vi "Open Session.vi"(0 "instruction target":refnum<class "niInstr Instruction Target v1 Host.lvclass">, 5 "parent context":refnum<class "niInstr Instruction Framework Context v1 Host.lvclass">, 7 "channel instance":u8, 11 "error in":errorcluster, 12 "select session":refnum<class "niHighSpeedSerial Eye Scan Single Point v1 Host.lvclass">) -> (4 "eye scan single point out":refnum<class "niHighSpeedSerial Eye Scan Single Point v1 Host.lvclass">, 15 "error out":errorcluster)   [LabVIEW 2016, in "niHighSpeedSerial Eye Scan Single Point v1 Host.lvclass"]
doc: "Opens a session to the Single Point Eye Scan class.\n\n<B>Input Parameters</B>\n\n<B>instruction target</B> is the instruction target to use when communicating with the FPGA.\n\n<B>parent context</B> is the context of the parent instance. In most cases you can wire a default value.\n\n<B>channel instance</B> The instance of the channel to be used.\n\n<B>error in</B> describes error conditions that occur before this node runs. This input provides standard 'error in' functionality.\n\n<B>Output Parameters</B>\n\n<B>eye scan single point out</B> passes a reference to your session to the next VI.\n\n<B>error out</B> contains error information. This output provides standard 'error out' functionality."
uses:
  <instrlib>/niHighSpeedSerial/Eye Scan/v1/Host/Impl/Single Point/niHighSpeedSerial Eye Scan Single Point v1 Host.lvclass
  <instrlib>/_niInstr/Instruction Framework/v1/Host/Instruction Target/niInstr Instruction Target v1 Host.lvclass
  <instrlib>/_niInstr/Instruction Framework/v1/Host/Instruction Framework Context/niInstr Instruction Framework Context v1 Host.lvclass
  <instrlib>/niHighSpeedSerial/Eye Scan/v1/Host/Impl/Single Point/Private/Private Data.ctl
  <instrlib>/niHighSpeedSerial/Register Maps/Xilinx/v1/Host/GTX2_CHANNEL v1 Host.llb/GTX2_CHANNEL Register Map.lvclass
  <instrlib>/niHighSpeedSerial/Eye Scan/v1/Host/Impl/Single Point/Private/Channel Measure State.ctl
  <instrlib>/niHighSpeedSerial/Eye Scan/v1/Host/Common/Public/Data Width.ctl
  <instrlib>/niHighSpeedSerial/Eye Scan/v1/Host/Common/Public/Point Offsets.ctl
  <instrlib>/niHighSpeedSerial/Register Maps/Xilinx/v1/Host/GTX2_CHANNEL v1 Host.llb/ESVertOffsetSign.ctl
  <instrlib>/niHighSpeedSerial/Eye Scan/v1/Host/Impl/Single Point/Private/Counts.ctl
  <instrlib>/niHighSpeedSerial/Register Maps/Xilinx/v1/Host/GTX2_CHANNEL v1 Host.llb/GTX2_CHANNEL Register Map.lvclass/GTX2_CHANNEL Register Map.ctl
  <instrlib>/niHighSpeedSerial/Eye Scan/v1/Host/Impl/Single Point/niHighSpeedSerial Eye Scan Single Point v1 Host.lvclass/niHighSpeedSerial Eye Scan Single Point v1 Host.ctl
  <instrlib>/_niInstr/Instruction Framework/v1/Host/Subsystem Map/Private/Lookup Single Context.vi
  <instrlib>/_niInstr/Instruction Framework/v1/Host/Subsystem Map/niInstr Subsystem Map v1 Host.lvclass
  <instrlib>/niHighSpeedSerial/Eye Scan/v1/Host/Common/niHighSpeedSerial Eye Scan Common v1 Host.lvlib
  <instrlib>/niHighSpeedSerial/Register Maps/Xilinx/v1/Host/GTX2_CHANNEL v1 Host.llb/GTX2_CHANNEL v1 Host.lvlib
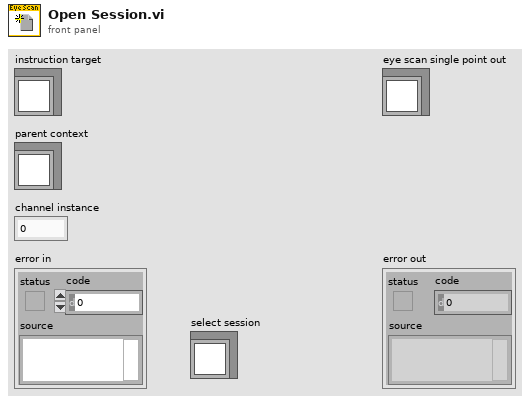
[diagram p1: front panel]
types:
  T1 = typedef "GTX2_CHANNEL v1 Host.lvlib/ESVertOffsetSign.ctl" = enum8{"Positive", "Negative"}
  T2 = typedef "niHighSpeedSerial Eye Scan Common v1 Host.lvlib/Data Width.ctl" = enum16{"16 Bit", "20 Bit", "32 Bit", "40 Bit"}
  T3 = typedef "niHighSpeedSerial Eye Scan Common v1 Host.lvlib/Point Offsets.ctl" = cluster{"horizontal offset":i16, "vertical offset":i8}
  T4 = typedef "niHighSpeedSerial Eye Scan Single Point v1 Host.lvclass/Channel Measure State.ctl" = enum16{"Uninitialized", "Initialized", "Ready", "Request", "Wait", "Read", "Process", "Finished"}
  T5 = typedef "niHighSpeedSerial Eye Scan Single Point v1 Host.lvclass/Private Data.ctl" = cluster{"GTX2_CHANNEL register map":refnum<class "GTX2_CHANNEL Register Map.lvclass">, "instruction target":refnum<class "niInstr Instruction Target v1 Host.lvclass">, "channel measure state":T4, "in DFE mode?":bool, "prescale":u8, "rx internal data width":T2, "active point":T3, "ut sign":T1, "positive counts":T6, "negative counts":T6}
  T6 = typedef "niHighSpeedSerial Eye Scan Single Point v1 Host.lvclass/Counts.ctl" = cluster{"sample count":u64, "error count":u16}
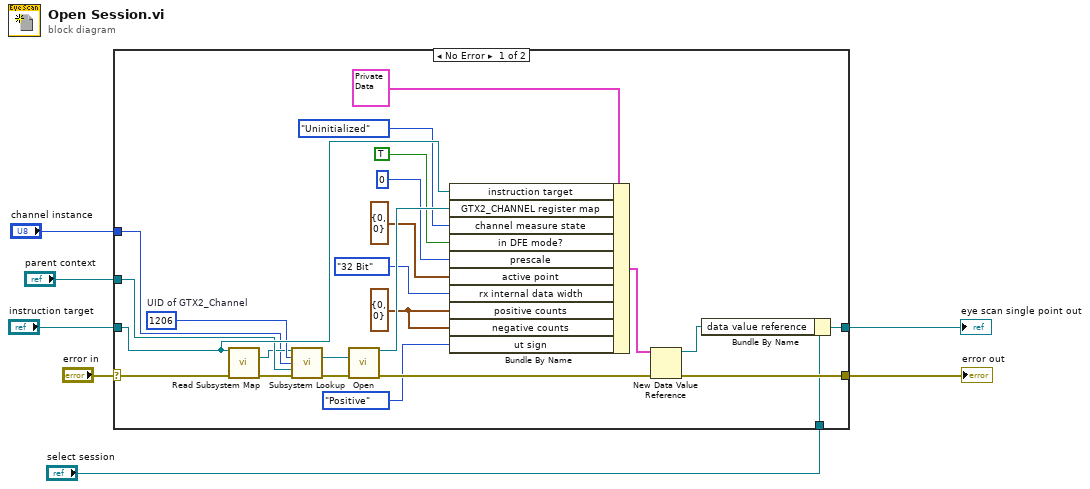
[diagram p0: block diagram]
diagram:
  n1 = case shown="No Error" "error in" {
    selector: "error in" -> [w16 w33]
    tunnel: [w18 w33] -> w6
    tunnel: [w17 w32] -> w1
    tunnel: "instruction target" -> [w28 _]
    tunnel: "parent context" -> [w27 _]
    tunnel: "channel instance" -> [w23 _]
    tunnel: "select session" -> [w8 w32]
    frame No Error {
      w9 = T6 {"sample count"=0, "error count"=0} ("positive counts")
      w26 = u16 1206  # UID of GTX2_Channel
      n2 = call <instrlib>:"Read Subsystem Map.vi"("instruction target in"=w28, "error in"=w16) -> ("subsystem map"=w24:refnum<class "niInstr Subsystem Map v1 Host.lvclass">, "error out"=w25:errorcluster)  [unwired: 11 in, 1 out]
      n3 = call-poly <instrlib>:"Subsystem Lookup.vi"("subsystem map in"=w24, "UID"=w26, "instance"=w23, "parent context (root)"=w27, "error in"=w25) -> ("context"=w22:refnum<class "niInstr Instruction Framework Context v1 Host.lvclass">, "error out"=w21:errorcluster)  [unwired: 7 in, 2 out]
      n4 = call <instrlib>:"Open.vi"("context"=w22, "error in"=w21) -> ("gtx2_channel register map object out"=w20:refnum<class "GTX2_CHANNEL Register Map.lvclass">, "error out"=w15:errorcluster)  [unwired: 12 in]
      n5 = Bundle By Name(cluster=T5 {"GTX2_CHANNEL register map"=refnum, "instruction target"=refnum, "channel measure state"=enum."Uninitialized", "in DFE mode?"=FALSE, "prescale"=0, "rx internal data width"=enum."32 Bit", "active point"={"horizontal offset"=0, "vertical offset"=0}, "ut sign"=enum."Positive", "positive counts"={"sample count"=0, "error count"=0}, "negative counts"={"sample count"=0, "error count"=0}} ("Private Data"), "instruction target"=w28, "GTX2_CHANNEL register map"=w20, "channel measure state"=Channel_Measure_State."Uninitialized" ("Measure State"), "in DFE mode?"=TRUE ("In DFE Mode?"), "prescale"=u8 0 ("Prescale"), "active point"=T3 {"horizontal offset"=0, "vertical offset"=0} ("Active Point"), "rx internal data width"=Data_Width."32 Bit" ("receiver data width"), "positive counts"=w9, "negative counts"=w9, "ut sign"=ESVertOffsetSign."Positive") -> (w30:T5)
      n6 = New Data Value Reference(data value=w30, error in=w15) -> (data value reference=w29:refnum<data-value>, error out=w18:errorcluster)
      n7 = Bundle By Name(cluster=w8, "data value reference"=w29) -> (w17:refnum<class "niHighSpeedSerial Eye Scan Single Point v1 Host.lvclass">)
    }
    frame Error {
    }
  }
  "error out" <- w6
  "eye scan single point out" <- w1
